vi "Serve.vi"(7 "Table in":refnum<class "Table.lvclass">, 8 "error in":errorcluster) -> (0 "error out":errorcluster, 5 "Table out":refnum<class "Table.lvclass">)   [LabVIEW 2021, in "Table.lvclass"]
uses:
  Table.lvclass
  Fork.ctl
  Hungry.ctl
  Philosopher/Philosopher.lvclass
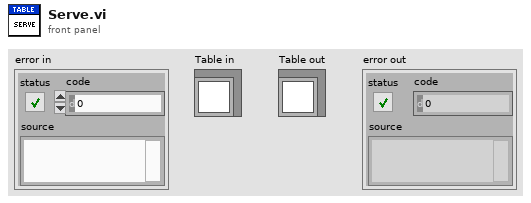
[diagram p1: front panel]
types:
  T1 = typedef "Table.lvclass/Hungry.ctl" = enum16{"NO", "YES"}
  T2 = typedef "Table.lvclass/Fork.ctl" = enum16{"FREE", "IN USE"}
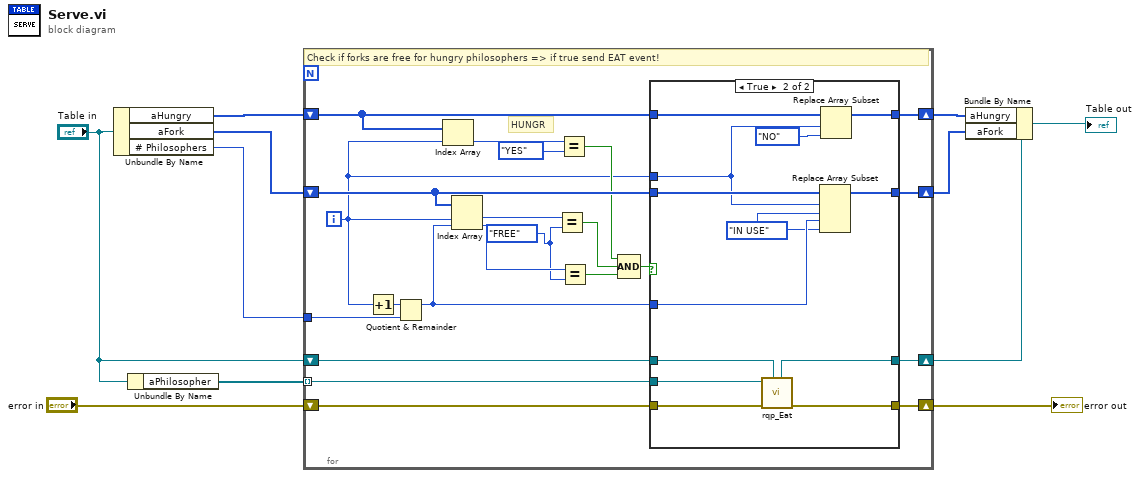
[diagram p0: block diagram]
diagram:
  n1 = Unbundle By Name("Table in") -> ("aHungry"=w11:T1[], "aFork"=w10:T2[], "# Philosophers"=w9:i32)
  n2 = Unbundle By Name("Table in") -> ("aPhilosopher"=w3:refnum<class "Philosopher.lvclass">[])
  n3 = for {
    tunnel: w9 -> [w32]
    shift-right: [w26] -> w6
    shift-left: w10 -> [w27]
    shift-right: [w22] -> w7
    shift-left: w11 -> [w23]
    shift-right: [w18] -> w8
    shift-left: "Table in" -> [w17]
    shift-right: [w15] -> w4
    shift-left: "error in" -> [w16]
    tunnel: w3 -> [w14] mode=indexing
    i -> [w21]
    w13 = Fork."FREE" ("Fork")
    # "HUNGR"
    # "Check if forks are free for hungry philosophers => if true send EAT event!"
    n4 = Increment(x=w21) -> (x+1=w33:i32)
    n5 = Quotient & Remainder(x=w33, y=w32) -> (x-y*floor(x/y)=w20:i32)  [unwired: 1 out]
    n6 = Index Array(array=w23, index=w21) -> (element=w25:T1)
    n7 = Index Array(array=w27, index #1=w21, index #2=w20) -> (element #1=w31:T2, element #2=w19:T2)
    n8 = Equal?(x=w31, y=w13) -> (x = y?=w29:bool)
    n9 = Equal?(x=w25, y=Hungry."YES" ("Hungry")) -> (x = y?=w24:bool)
    n10 = Equal?(x=w19, y=w13) -> (x = y?=w30:bool)
    n11 = Compound Arithmetic op=AND(w24, w29, w30) -> (w28:bool)
    n12 = case shown="True" w28 {
      tunnel: w27 -> [w37 w50]
      tunnel: w21 -> [_ w48]
      tunnel: w20 -> [_ w46]
      tunnel: [w37 w45] -> w26
      tunnel: w23 -> [w36 w49]
      tunnel: [w36 w47] -> w22
      tunnel: [w35 w39] -> w18
      tunnel: w17 -> [w35 w38]
      tunnel: w16 -> [w34 w41]
      tunnel: [w34 w42] -> w15
      tunnel: w14 -> [_ w40]
      frame False {
      }
      frame True {
        w44 = Fork."IN USE" ("Fork")
        n13 = call "rqp_Eat.vi"("Caller in"=w38, "error in"=w41, "Philosopher in"=w40) -> ("error out"=w42:errorcluster, "dup Caller out"=w39:refnum<class "Table.lvclass">)  [unwired: 6 in, 1 out]
        n14 = Replace Array Subset(array=w50, new element #1=w44, index #1=w48, new element #2=w44, index #2=w46) -> (w45:T2[])
        n15 = Replace Array Subset(array=w49, new element=Hungry."NO" ("Hungry"), index=w48) -> (w47:T1[])
      }
    }
  }
  "error out" <- w4
  n16 = Bundle By Name(cluster=w8, "aHungry"=w7, "aFork"=w6) -> (→"Table out":refnum<class "Table.lvclass">)
